vi "Day 4.2 - Total scratchcards.vi"(11 "input":string[](array[string])) -> (3 "ouptut part 2":u64)   [LabVIEW 2021]
panel:
  out "Game":u32[][](array[numeric])
  out "Winning Nos":u32[][](array[numeric])
  out "Winning Scores":u32[](array[numeric])
  out "Card":i32
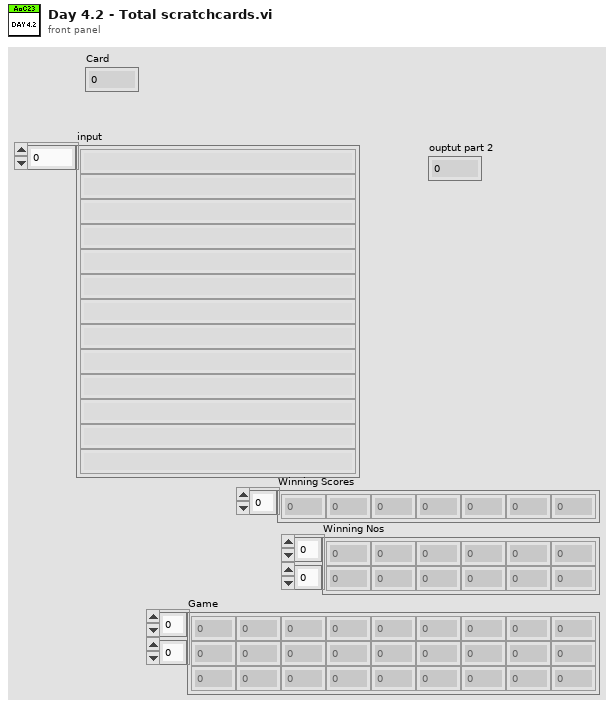
[diagram p1: front panel]
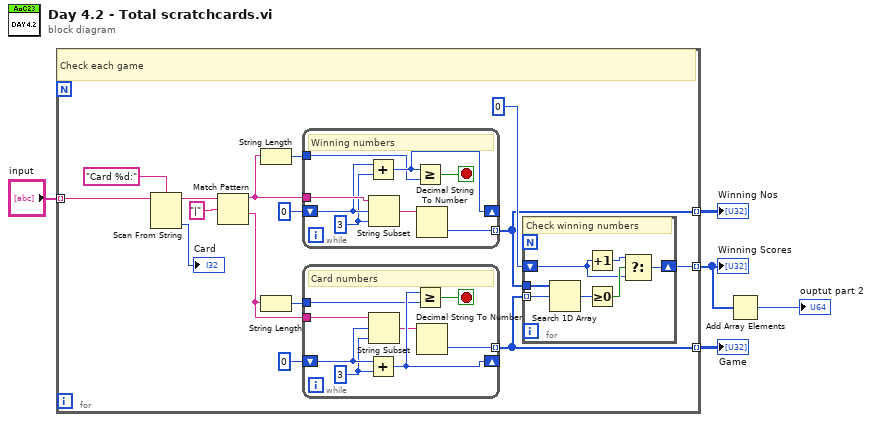
[diagram p0: block diagram]
diagram:
  n1 = for {
    tunnel: "input" -> [w20] mode=indexing
    tunnel: [w14] -> w5 mode=indexing
    tunnel: [w10] -> w4 mode=indexing
    tunnel: [w6] -> w3 mode=indexing
    # "Check each game"
    n2 = Scan From String(format string="Card %d:", input string=w20) -> (remaining string=w17:string, output 1=→"Card":i32)  [unwired: 3 in, 2 out]
    n3 = Match Pattern(string=w17, regular expression="|") -> (before substring=w12:string, after substring=w7:string)  [unwired: 1 in, 2 out]
    n4 = String Length(string=w12) -> (length=w11:i32)
    n5 = String Length(string=w7) -> (length=w9:i32)
    n6 = while {
      tunnel: w12 -> [w36]
      shift-right: [w32] -> _
      shift-left: 0 -> [w34]
      tunnel: w11 -> [w31]
      tunnel: [w29] -> w10 mode=indexing
      stop <- w35 stop-if-true
      w33 = 3 ("length (rest)")
      # "Winning numbers"
      n7 = Add(x=w34, y=w33) -> (x+y=w32:i32)
      n8 = String Subset(string=w36, offset (0)=w34, length (rest)=w33) -> (substring=w30:string)
      n9 = Greater Or Equal?(x=w32, y=w31) -> (x >= y?=w35:bool)
      n10 = Decimal String To Number(string=w30) -> (number=w29:i32)  [unwired: 2 in, 1 out]
    }
    n11 = while {
      tunnel: w7 -> [w28]
      shift-right: [w24] -> _
      shift-left: 0 -> [w26]
      tunnel: w9 -> [w23]
      tunnel: [w21] -> w6 mode=indexing
      stop <- w27 stop-if-true
      w25 = 3 ("length (rest)")
      # "Card numbers"
      n12 = Add(x=w26, y=w25) -> (x+y=w24:i32)
      n13 = String Subset(string=w28, offset (0)=w26, length (rest)=w25) -> (substring=w22:string)
      n14 = Greater Or Equal?(x=w24, y=w23) -> (x >= y?=w27:bool)
      n15 = Decimal String To Number(string=w22) -> (number=w21:i32)  [unwired: 2 in, 1 out]
    }
    n16 = for {
      tunnel: w6 -> [w42] mode=indexing
      tunnel: w10 -> [w43]
      shift-right: [w39] -> w14
      shift-left: 0 -> [w37]
      # "Check winning numbers"
      n17 = Search 1D Array(1D array=w43, element=w42) -> (index of element=w41:i32)  [unwired: 1 in]
      n18 = Increment(x=w37) -> (x+1=w38:i32)
      n19 = Greater Or Equal To 0?(x=w41) -> (x >= 0?=w40:bool)
      n20 = Select(t=w38, s=w40, f=w37) -> (s? t:f=w39:i32)
    }
  }
  "Winning Scores" <- w5
  "Winning Nos" <- w4
  "Game" <- w3
  n21 = Add Array Elements(numeric array=w5) -> (sum=→"ouptut part 2":i32)
